vi "readFromXML.vi"(8 "error in (no error)":errorcluster, 10 "XML in":string, 11 "StartUp in":refnum<class "StartUp.lvclass">) -> (0 "error out":errorcluster, 3 "StartUp out":refnum<class "StartUp.lvclass">)   [LabVIEW 2014, in "TCSDataDefinitions.lvlib" / "TCSCommand.lvlib" / "StartUp.lvclass"]
uses:
  StartUp.lvclass
  TCSTcsCommand/TCSTcsCommand.lvclass
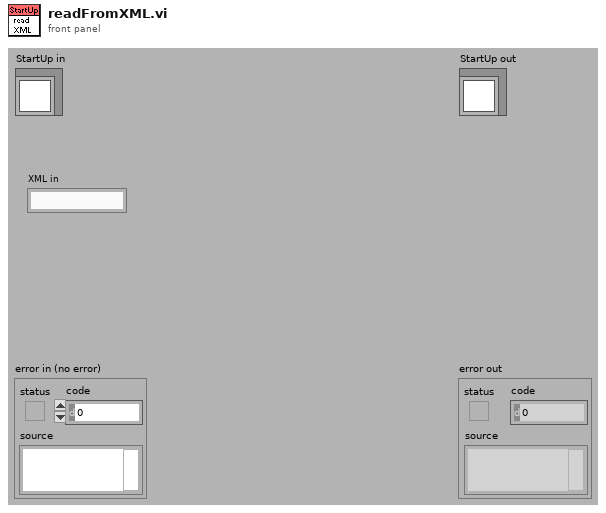
[diagram p1: front panel]
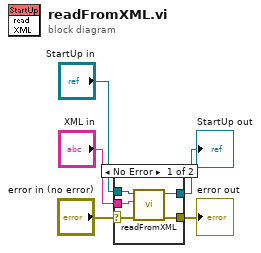
[diagram p0: block diagram]
diagram:
  n1 = case shown="No Error" "error in (no error)" {
    selector: "error in (no error)" -> [w6 w12]
    tunnel: [w10 w12] -> w5
    tunnel: [w9 w11] -> w4
    tunnel: "XML in" -> [w8 _]
    tunnel: "StartUp in" -> [w7 w11]
    frame No Error {
      n2 = call-parent "readFromXML.vi"("error in (no error)"=w6, "XMLin"=w8, "TCSTcsCommand in"=w7) -> ("error out"=w10:errorcluster, "TCSTcsCommand out"=w9:refnum<class "StartUp.lvclass">)  [unwired: 7 out]
    }
    frame Error {
    }
  }
  "error out" <- w5
  "StartUp out" <- w4
